vi "DMR_ImageRequestSingle.vi"(4 "request control IN":i32, 5 "driver handle IN":i32) -> (0 "error code OUT":i32, 1 "request used OUT":i32, 2 "driver handle OUT":i32)   [LabVIEW 2014]
doc: "Sends an image request to the device driver.\n\nThis functions sends a single image request to the camera. To wait for the image\nto become ready call the VI DMR_ImageRequestWaitFor.\n\nNote:\nIn order to make sure, that no image data is lost it is important to understand, how the request mechanism works. The driver works with a fixed number of request objects. The number of request objects available to the driver can be set by modifying the value of the property 'RequestCount' in the system list.\n\nEach request will consum a certain amount of memory. Once an image has been captured by the request this amount will be slightly more then the image itself needs in memory, so modify this parameter gently.\n\nOn the other hand it's neccessary to have more then a single request in order to ensure a lossless acquisition. E.g. when working with free running cameras image might be lost because when an image has been captured and processed the next vertical sync. pulse has already been missed when the request is unlocked again.\n\nSee also:\nDMR_ImageRequestReset,\nDMR_ImageRequestUnlock,\nDMR_ImageRequestWaitFor\n\nThe 'error code OUT' terminal will deliver 0 if successful or a negative error code otherwise. A list of valid error codes and their meaning can be found in the manual about this interface."
uses:
  mvDeviceManager.dll
panel:
  # "OUTPUT"
  # "INPUT"
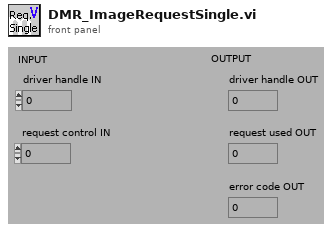
[diagram p1: front panel]
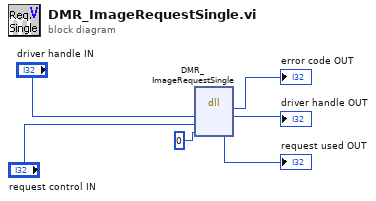
[diagram p0: block diagram]
diagram:
  n1 = dll-call lib="mvDeviceManager.dll" fn="DMR_ImageRequestSingle"("hDrv"="driver handle IN", "requestCtrl"="request control IN", "pRequestUsed"=0) -> (→"error code OUT":i32, "hDrv"=→"driver handle OUT":i32, "pRequestUsed"=→"request used OUT":i32)  [unwired: 4 in, 2 out]
